vi "process data files.vi"(11 "makeSpeedlinesData in":T1) -> (1 "appended array":cluster{"mDot":dbl[], "PR":dbl[]}[](array[cluster]), 3 "makeSpeedlinesData out":T1)   [LabVIEW 2018]
uses:
  make speedlines UI data.ctl
  <vilib>/Analysis/baseanly.llb/Mean (DBL).vi
  <vilib>/Analysis/NI_AALBase.lvlib
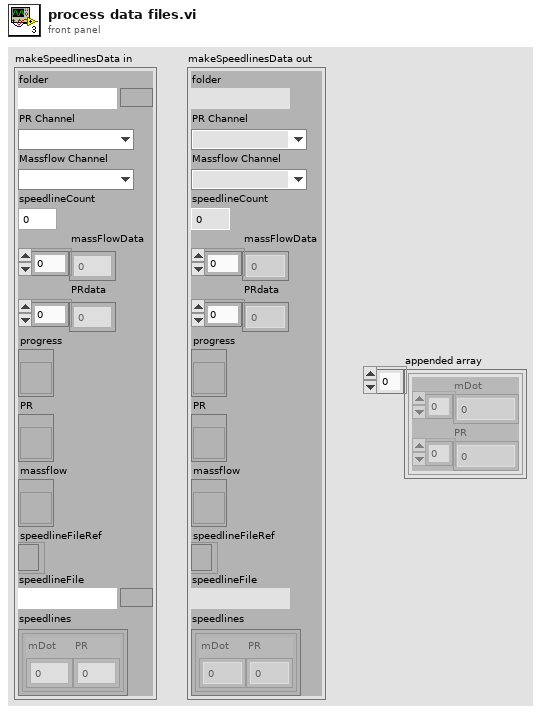
[diagram p1: front panel]
types:
  T1 = typedef "make speedlines UI data.ctl" = cluster{"folder":path, "PR Channel":u16, "Massflow Channel":u16, "speedlineCount":u16, "massFlowData":dbl[], "PRdata":dbl[], "progress":refnum<vi>, "PR":refnum<vi>, "massflow":refnum<vi>, "speedlineFileRef":refnum<file>, "speedlineFile":path, "speedlines":cluster{"mDot":dbl[], "PR":dbl[]}[]}
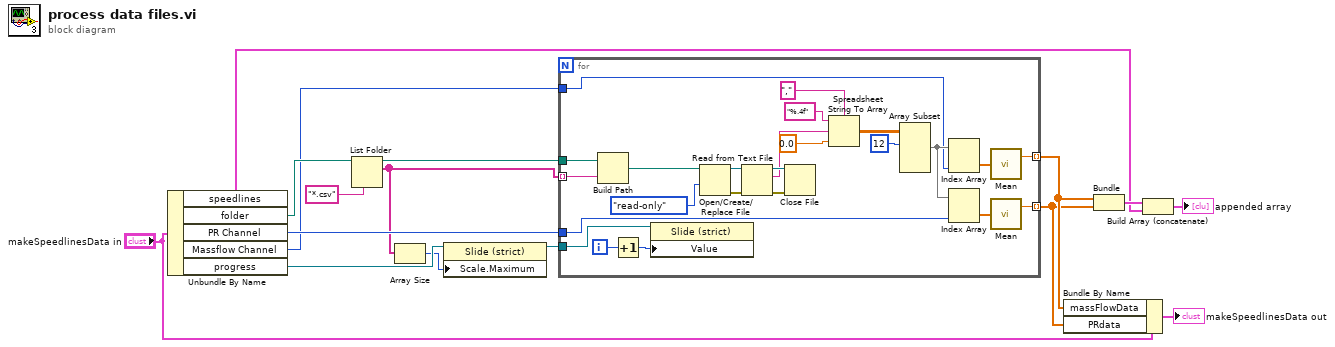
[diagram p0: block diagram]
diagram:
  n1 = Unbundle By Name("makeSpeedlinesData in") -> ("speedlines"=w2:cluster{"mDot":dbl[], "PR":dbl[]}[], "folder"=w14:path, "PR Channel"=w11:u16, "Massflow Channel"=w10:u16, "progress"=w6:refnum<vi>)
  n2 = List Folder(path=w14, pattern="*.csv") -> (path out=w12:path, filenames=w5:string[])  [unwired: 2 in, 2 out]
  n3 = Array Size(array=w5) -> (size(s)=w4:i32)
  n4 = property class="Slide (strict)"(reference=w6, "Scale.Maximum"=w4) -> (reference out=w3:refnum<vi>)  [unwired: 1 in, 1 out]
  n5 = for {
    tunnel: w5 -> [w39] mode=indexing
    tunnel: w12 -> [w40]
    tunnel: w11 -> [w28]
    tunnel: w10 -> [w27]
    tunnel: [w24] -> w8 mode=indexing
    tunnel: [w23] -> w9 mode=indexing
    tunnel: w3 -> [w22]
    i -> [w21]
    n6 = Build Path(base path=w40, name or relative path=w39) -> (appended path=w38:path)
    n7 = Increment(x=w21) -> (x+1=w20:i32)
    n8 = property class="Slide (strict)"(reference=w22, "Value"=w20) -> ()  [unwired: 1 in, 2 out]
    n9 = Open/Create/Replace File(file path (use dialog)=w38, access (0:read/write)=enum16{"read/write", "read-only", "write-only"}."read-only") -> (refnum out=w35:refnum<file>, error out=w36:errorcluster)  [unwired: 4 in, 1 out]
    n10 = Read from Text File(file (use dialog)=w35, error in=w36) -> (refnum out=w33:refnum<file>, text=w18:string, error out=w34:errorcluster)  [unwired: 2 in, 1 out]
    n11 = Close File(refnum=w33, error in=w34) -> ()  [unwired: 2 out]
    n12 = Spreadsheet String To Array(delimiter (Tab)=",", format string="%.4f" ("spreadsheet string"), spreadsheet string=w18, array type (2D Dbl)=0.0) -> (array=w31:dbl[][])
    n13 = Array Subset(array=w31, index (row)=12 ("index")) -> (w29:dbl[][])  [unwired: 3 in]
    n14 = Index Array(array=w29, index (col)=w27) -> (element=w25:dbl[])  [unwired: 1 in]
    n15 = Index Array(array=w29, index (col)=w28) -> (element=w26:dbl[])  [unwired: 1 in]
    n16 = call-poly <vilib>:"Mean.vi"("X"=w25) -> ("mean"=w23:dbl)  [unwired: 1 out]
    n17 = call-poly <vilib>:"Mean.vi"("X"=w26) -> ("mean"=w24:dbl)  [unwired: 1 out]
  }
  n18 = Bundle By Name(cluster="makeSpeedlinesData in", "massFlowData"=w9, "PRdata"=w8) -> (→"makeSpeedlinesData out":T1)
  n19 = Bundle(w9, w8) -> (w7:cluster{dbl[], dbl[]})  [unwired: 1 in]
  n20 = Build Array (concatenate)(w7, w2) -> (→"appended array":cluster{"mDot":dbl[], "PR":dbl[]}[])
